vi "Message over the network.vi"(0 "Guardian in":refnum<class "Guardian.lvclass">, 1 "Destination GD ID":string, 2 "Target ID (uService ID or \"Guardian\")":string, 3 "Message":string, 4 "Data":variant, 5 "error in (no error)":errorcluster) -> (14 "Guardian out":refnum<class "Guardian.lvclass">, 19 "error out":errorcluster)   [LabVIEW 2026, in "TALOS.lvlib" / "Guardian.lvlib" / "Guardian.lvclass"]
doc: "To send a message to a Guardian, type \"Guardian\" into the Target ID field."
uses:
  Guardian.lvclass
  Guardian.lvclass/Guardian.ctl
  Internal uServices/System uServices/TCP Writer/TCP Writer/TCP Message Internal Composition.ctl
  Ancestor/Ancestor/Ancestor.lvclass/Ancestor.ctl
  Support VIs/Generate Error.vi
  FGV/Error Memory/Get Error Description.vi
  Support VIs/Get PC name.vi
  Ancestor/Ancestor/Read ID.vi
  Support VIs/Get Class Name.vi
  <vilib>/Utility/error.llb/Clear Errors.vi
  FGV/Error Memory/Error Memory Core.vi
  <vilib>/AdvancedString/Delimited String to 1D String Array.vi
  <vilib>/AdvancedString/Delimited String to 1D String Array (string).vi
  Support VIs/Circus Root Path.vi
  FGV/Error Memory/Error Crt Lvl checker.vi
  FGV/Error Memory/Error Memory Core.vi/40c8088d-b597-4017-91af-faa98e00292e.vi
  FGV/Error Memory/Error Memory Core.vi/d4a3ab98-063c-4e44-b43d-fbdcfe6c2be2.vi
  Support VIs/Global Memory.vi
  <vilib>/Utility/LVClass/Get LV Class Name.vi
  Support VIs/Is in Packed Library.vi
  Support VIs/TALOS Root path.vi
  Support VIs/Read CSV worksheet.vi
  Support VIs/Global Constants.vi
  <vilib>/Utility/error.llb/General Error Handler.vi
  Support VIs/Error Log.vi
  Ancestor/Ancestor/Ancestor.lvclass
  <vilib>/Comparison/Equal/Equal Functor/Equal Functor.lvclass
  Classes/Guardian List/Guardian List.lvclass
  Internal uServices/System uServices/TCP Writer/TCP Writer/TCP Writer.lvclass
  TALOS.lvlib
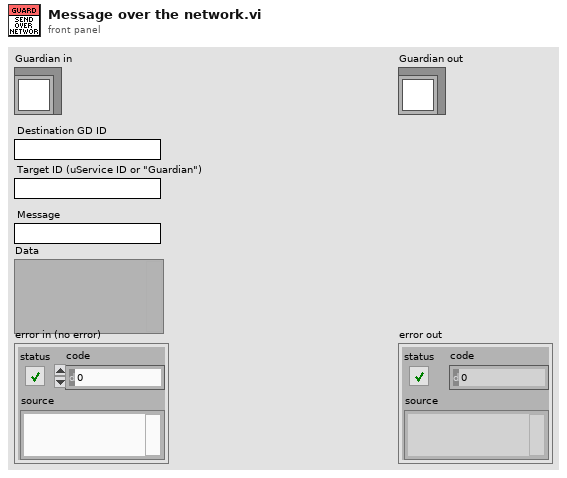
[diagram p1: front panel]
types:
  T1 = typedef "TALOS.lvlib/TCP Writer.lvlib/TCP Writer.lvclass/TCP Message Internal Composition.ctl" = cluster{"uS/GD ID":string, "Message":string, "Data":variant}
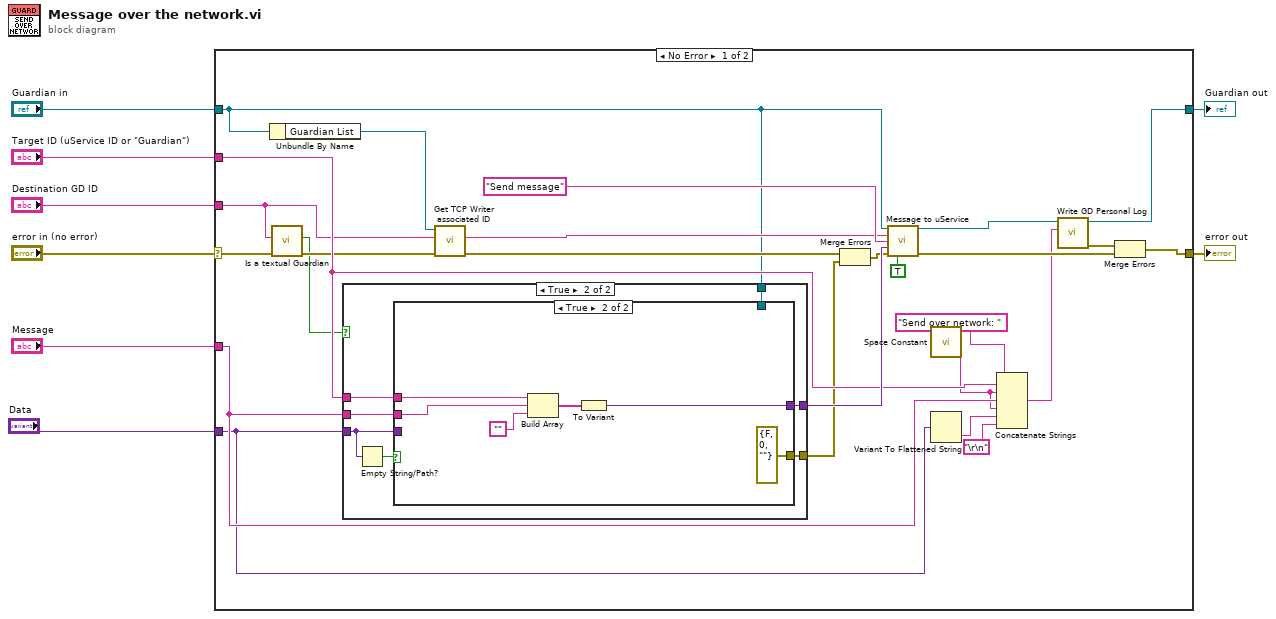
[diagram p0: block diagram]
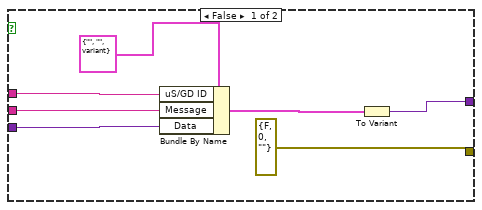
[diagram p2: hidden frame]
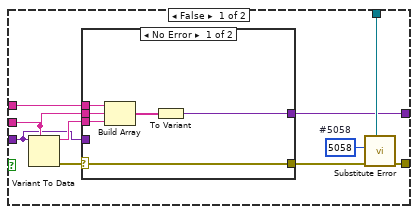
[diagram p3: hidden frame]
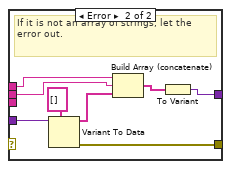
[diagram p4: hidden frame]
diagram:
  n1 = case shown="No Error" "error in (no error)" {
    selector: "error in (no error)" -> [w15 w80]
    tunnel: [w25 w80] -> w8
    tunnel: "Guardian in" -> [w11 w79]
    tunnel: "Data" -> [w20 _]
    tunnel: "Message" -> [w21 _]
    tunnel: "Target ID (uService ID or \"Guardian\")" -> [w22 _]
    tunnel: "Destination GD ID" -> [w14 _]
    tunnel: [w27 w79] -> w1
    frame No Error {
      n2 = Unbundle By Name(w11) -> ("Guardian List"=w29:refnum<class "Guardian List.lvclass">)
      n3 = call "Is a textual Guardian.vi"("error in (no error)"=w15, "Target GD ID"=w14) -> ("error out"=w13:errorcluster, "Textual?"=w12:bool)  [unwired: 8 in]
      n4 = case shown="True" w12 {
        tunnel: [w36 w44] -> w33
        tunnel: w22 -> [w39 w46]
        tunnel: w21 -> [w38 w45]
        tunnel: w20 -> [w37 w43]
        tunnel: w11 -> [_ w48]
        tunnel: [errorcluster {"status"=FALSE, "code"=0, "source"=""} ("error out") w47] -> w9
        frame False {
          n5 = Bundle By Name(cluster=T1 {"uS/GD ID"="", "Message"="", "Data"=variant}, "uS/GD ID"=w39, "Message"=w38, "Data"=w37) -> (w41:T1)
          n6 = To Variant(anything=w41) -> (Variant=w36:variant)
        }
        frame True {
          n7 = Empty String/Path?(string/path=w43) -> (empty?=w42:bool)
          n8 = case shown="True" w42 {
            tunnel: w48 -> [w57 _]
            tunnel: [w56 errorcluster {"status"=FALSE, "code"=0, "source"=""} ("error out")] -> w47
            tunnel: w46 -> [w55 w77]
            tunnel: w45 -> [w54 w76]
            tunnel: [w53 w74] -> w44
            tunnel: w43 -> [w49 _]
            frame False {
              w58 = 5058  # #5058
              n9 = Variant To Data(type=w54, Variant=w49) -> (data=w52:string, error out=w51:errorcluster)  [unwired: 1 in]
              n10 = case shown="No Error" w51 {
                selector: w51 -> [w59 _]
                tunnel: w55 -> [w64 w69]
                tunnel: w54 -> [w63 w68]
                tunnel: [w61 w65] -> w53
                tunnel: w52 -> [w60 _]
                tunnel: [w59 w70] -> w50
                tunnel: w49 -> [_ w72]
                frame No Error {
                  n11 = Build Array(w64, w63, w60) -> (w62:string[])
                  n12 = To Variant(anything=w62) -> (Variant=w61:variant)
                }
                frame Error {
                  # "If it is not an array of strings, let the error out."
                  n13 = Variant To Data(type=string[] [], Variant=w72) -> (data=w67:string[], error out=w70:errorcluster)  [unwired: 1 in]
                  n14 = Build Array (concatenate)(w69, w68, w67) -> (w66:string[])
                  n15 = To Variant(anything=w66) -> (Variant=w65:variant)
                }
              }
              n16 = call "Substitute Error.vi"("LabVIEW Object"=w57, "error in (no error)"=w50, "Error Code"=w58) -> ("error out"=w56:errorcluster)  [unwired: 8 in]
            }
            frame True {
              n17 = Build Array(w77, w76, "") -> (w78:string[])
              n18 = To Variant(anything=w78) -> (Variant=w74:variant)
            }
          }
        }
      }
      n19 = call-dynamic "Get TCP Writer associated ID.vi"("error in (no error)"=w13, "ID"=w14, "Guardian List in"=w29) -> ("error out"=w30:errorcluster, "TCP Writer associated ID"=w31:string)  [unwired: 6 in, 1 out]
      n20 = Merge Errors(w30, w9) -> (w10:errorcluster)
      n21 = call "Message to uService.vi"("Guardian in"=w11, "uService ID"=w31, "Message"="Send message" ("Item Name"), "Data"=w33, "error in (no error)"=w10, "Locale?"=TRUE) -> ("Guardian out"=w28:refnum<class "Guardian.lvclass">, "error out"=w24:errorcluster)  [unwired: 8 in]
      n22 = call <vilib>:"Space Constant.vi"() -> ("String"=w17:string)
      n23 = Variant To Flattened String(Variant=w20) -> (data string=w19:string)  [unwired: 1 out]
      n24 = Concatenate Strings("Send over network: " ("string"), w22, w17, w21, w17, w19, "\r\n") -> (w18:string)
      n25 = call "Write GD Personal Log.vi"("String"=w18, "Guardian in"=w28) -> ("error out"=w26:errorcluster, "Guardian out"=w27:refnum<class "Guardian.lvclass">)  [unwired: 8 in]
      n26 = Merge Errors(w26, w24) -> (w25:errorcluster)
    }
    frame Error {
    }
  }
  "error out" <- w8
  "Guardian out" <- w1
